vi "Initialize_Control.vi"(0 "GEA2":refnum<queue>, 1 "ERD Loop":refnum<queue>, 5 "Receive Loop Error":refnum<user-event>, 7 "UI Loop Error":refnum<user-event>, 9 "DAQ":refnum<queue>, 11 "Error In":errorcluster, 12 "Cont Send":T1) -> (15 "Error Out":errorcluster)   [LabVIEW 2014]
uses:
  type defs/DAQ_States.ctl
  type defs/ERD_Data_Loop_Control.ctl
  Utility/Labview GEA2 Toolkit v2.1/GExplorer Support/typedefs/GExplorer_Data_Cluster.ctl
  type defs/Ref_Cont_Send_Queue.ctl
  type defs/Cont_Send_States.ctl
  type defs/Error_Command.ctl
  type defs/ERD_Loop_Control_Command.ctl
  type defs/GEA2_Control_Command.ctl
  type defs/DAQ_Control_Command.ctl
  type defs/Cont_Send_Loop_Control_Command.ctl
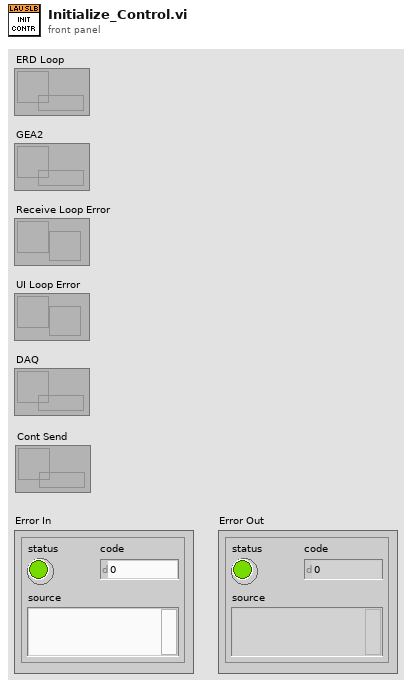
[diagram p1: front panel]
types:
  T1 = typedef "Ref_Cont_Send_Queue.ctl" = refnum<queue>
  T2 = typedef "Cont_Send_Loop_Control_Command.ctl" = enum16{"Initialize", "Shutdown"}
  T3 = typedef "DAQ_Control_Command.ctl" = enum16{"Initialize", "Shutdown"}
  T4 = typedef "GEA2_Control_Command.ctl" = enum16{"Initialize", "Shutdown"}
  T5 = typedef "ERD_Loop_Control_Command.ctl" = enum16{"Initialize", "Shutdown"}
  T6 = typedef "Error_Command.ctl" = enum16{"Initialize", "Handle Errors", "Report Errors"}
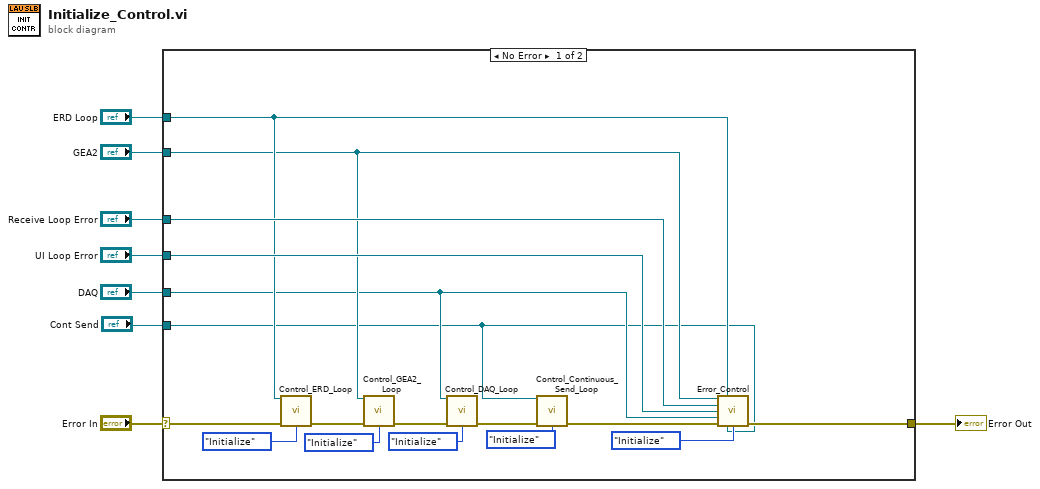
[diagram p0: block diagram]
diagram:
  n1 = case shown="No Error" "Error In" {
    selector: "Error In" -> [w21 w26]
    tunnel: [w25 w26] -> w7
    tunnel: "Receive Loop Error" -> [w24 _]
    tunnel: "ERD Loop" -> [w20 _]
    tunnel: "GEA2" -> [w17 _]
    tunnel: "UI Loop Error" -> [w22 _]
    tunnel: "DAQ" -> [w14 _]
    tunnel: "Cont Send" -> [w9 _]
    frame No Error {
      n2 = call "Control_ERD_Loop.vi"("ERD Loop"=w20, "Command (ERD Loop Control)"=ERD_Loop_Control_Command."Initialize", "Error In"=w21) -> ("Error Out"=w18:errorcluster)  [unwired: 12 in]
      n3 = call "Control_GEA2_Loop.vi"("GEA2"=w17, "Command (ERD Loop Control)"=GEA2_Control_Command."Initialize", "Error In"=w18) -> ("Error Out"=w15:errorcluster)  [unwired: 12 in]
      n4 = call "Control_DAQ_Loop.vi"("DAQ"=w14, "Command (DAQ Control)"=DAQ_Control_Command."Initialize" ("Command (DAQ)"), "Error In"=w15) -> ("Error Out"=w12:errorcluster)  [unwired: 12 in]
      n5 = call "Control_Continuous_Send_Loop.vi"("Cont Send"=w9, "Cont Send Loop Control Command"=Cont_Send_Loop_Control_Command."Initialize", "Error In"=w12) -> ("Error Out"=w11:errorcluster)  [unwired: 12 in]
      n6 = call "Error_Control.vi"("GEA2"=w17, "ERD Loop"=w20, "Command (Handle Errors)"=Error_Command."Initialize", "Receive Loop Error"=w24, "UI Loop Error"=w22, "DAQ"=w14, "Error In"=w11, "Cont Send"=w9) -> ("Error Out"=w25:errorcluster)  [unwired: 7 in]
    }
    frame Error {
    }
  }
  "Error Out" <- w7
